vi "PixyGetFrame.vi"() -> (3 "Frame":string)   [LabVIEW 2016]
uses:
  <vilib>/regexp/Match Regular Expression.xnode
panel:
  out "error out":errorcluster
  out "Pixy Data":string
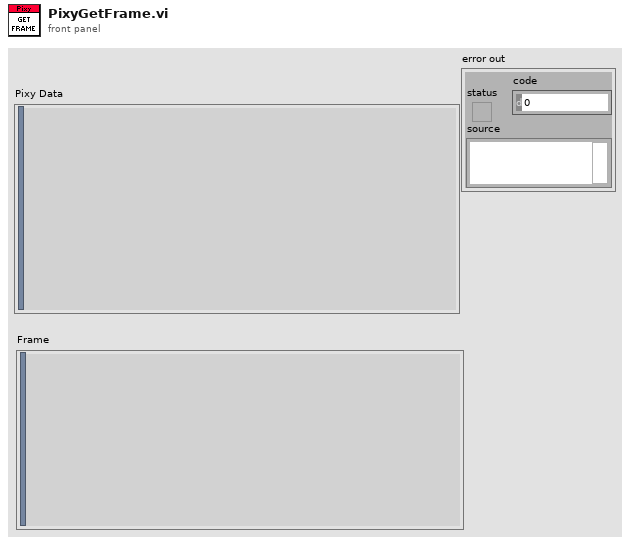
[diagram p1: front panel]
types:
  T1 = typedef "WPI_I2CDevRef.ctl" = cluster{"DevStatus":errorcluster, "Device Address":u8, "Handle":i32, "I2C Bus":T2}
  T2 = typedef "i2c_bus.ctl" = enum16{"I2C On-Board", "I2C MXP", "Invalid"}
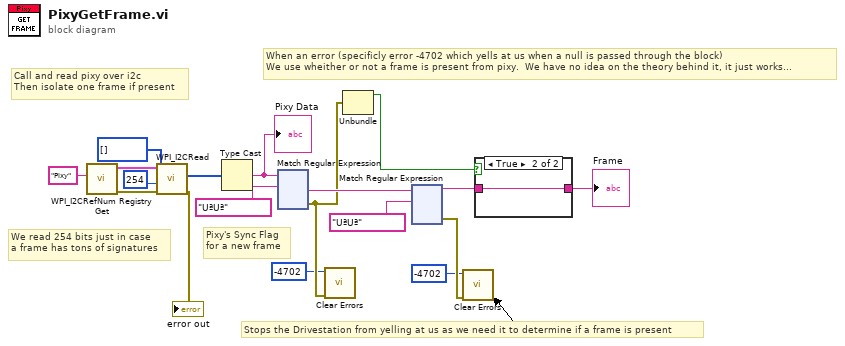
[diagram p0: block diagram]
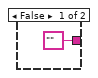
[diagram p2: hidden frame]
diagram:
  # "Pixy's Sync Flag\nfor a new frame"
  # "We read 254 bits just in case\na frame has tons of signatures"
  # "Stops the Drivestation from yelling at us as we need it to determine if a frame is present"
  # "When an error (specificly error -4702 which yells at us when a null is passed through the block)\nWe use wheither or not a frame is present from pixy.  We have no idea on the theory behind it, it just works..."
  # "Call and read pixy over i2c\nThen isolate one frame if present"
  n1 = call <vilib>:"WPI_I2CRefNum Registry Get.vi"("refnum name"="Pixy") -> ("error out"=w17:errorcluster, "I2CDevRef"=w16:T1)  [unwired: 9 in]
  n2 = call <vilib>:"WPI_I2CRead.vi"("error in (no error)"=w17, "I2CBytesToRead"=u8 254, "I2CRegister"=u8[] [], "I2CDevRef"=w16) -> ("error out"=→"error out":errorcluster, "Data Out"=w13:u8[])  [unwired: 5 in, 1 out]
  n3 = Type Cast(x=w13) -> (*(type *) &x=w9:string)  [unwired: 1 in]
  "Pixy Data" <- w9
  n4 = xnode "Match Regular Expression"("input string"=w9, "regular expression"="UªUª") -> ("after match"=w10:string, "error out"=w5:errorcluster)  [unwired: 4 in, 3 out]
  n5 = call <vilib>:"Clear Errors.vi"("error in (no error)"=w5, "specific error code to clear (0: all)"=-4702) -> ()  [unwired: 4 in, 2 out]
  n6 = Unbundle(w5) -> ("status"=w8:bool)  [unwired: 2 out]
  n7 = xnode "Match Regular Expression"("input string"=w10, "regular expression"="UªUª") -> ("before match"=w6:string, "error out"=w3:errorcluster)  [unwired: 4 in, 3 out]
  n8 = call <vilib>:"Clear Errors.vi"("error in (no error)"=w3, "specific error code to clear (0: all)"=-4702) -> ()  [unwired: 4 in, 2 out]
  n9 = case shown="True" w8 {
    tunnel: ["" ("before match") w20] -> w7
    tunnel: w6 -> [_ w20]
    frame False {
    }
    frame True {
    }
  }
  "Frame" <- w7
